vi "ChipKit Blink.vi"() -> ()   [LabVIEW 2011, in "LabVIEW Interface for ChipKit.lvlib"]
uses:
  vi.lib/LabVIEW Interface for ChipKit/LabVIEW Interface for ChipKit.lvlib
  vi.lib/LabVIEW Interface for ChipKit/Private/Type Defs/Board Type.ctl
  vi.lib/LabVIEW Interface for ChipKit/Private/Type Defs/Chipkit Resource.ctl
  vi.lib/LabVIEW Interface for ChipKit/Private/Type Defs/Analog Pin.ctl
panel:
  in  "Analog Pin":T1=enum."AI_12"
  in  "ChipKit Configuration":T2={"VISA resource"="COM3", "Board Type"=enum."Arduino Uno", "Connection Type"=enum."USB / Serial", "Bytes Per Packet (15)"=0}
  in  "Stop Button":bool
  out "Voltage":dbl
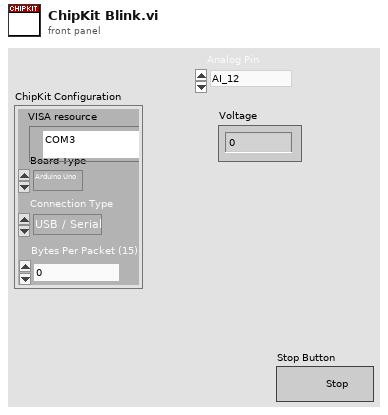
[diagram p1: front panel]
types:
  T1 = typedef "LabVIEW Interface for ChipKit.lvlib/Analog Pin.ctl" = enum8{"AI_0", "AI_1", "AI_2", "AI_3", "AI_4", "AI_5", "AI_6", "AI_7", "AI_8", "AI_9", "AI_10", "AI_11", "AI_12", "AI_13", "AI_14", "AI_15"}
  T2 = typedef "LabVIEW Interface for ChipKit.lvlib/Chipkit Resource.ctl" = cluster{"VISA resource":refnum<visa-resource-name>, "Board Type":T3, "Connection Type":enum8{"USB / Serial"}, "Bytes Per Packet (15)":u8}
  T3 = typedef "LabVIEW Interface for ChipKit.lvlib/Board Type.ctl" = enum16{"Arduino Uno", "Dimuelanove w/Atmega 328", "Mega 2560", "Chipkit Uno32", "Chipkit Max32"}
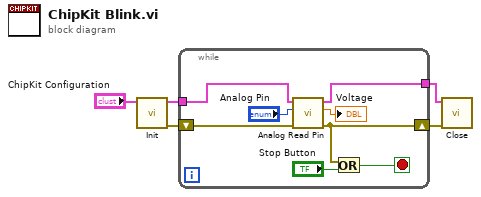
[diagram p0: block diagram]
diagram:
  n1 = call "Init.vi"("ChipKit Configuration"="ChipKit Configuration") -> ("Error Out"=w3:errorcluster, "ChipKit Configuration"=w5:T2)  [unwired: 9 in]
  n2 = while {
    tunnel: w5 -> [w13]
    tunnel: [w12] -> w4
    shift-right: [w9] -> w2
    shift-left: w3 -> [w10]
    stop <- w7 stop-if-true
    n3 = call "Analog Read Pin.vi"("Error In"=w10, "Analog Pin"="Analog Pin", "ChipKit Resource"=w13) -> ("Error Out"=w9:errorcluster, "Voltage"=→"Voltage":dbl, "ChipKit Resource"=w12:T2)  [unwired: 6 in]
    n4 = Or(x=w9, y="Stop Button") -> (x .or. y?=w7:bool)
  }
  n5 = call "Close.vi"("Error In"=w2, "ChipKit Configuration"=w4) -> ()  [unwired: 9 in, 1 out]
